vi "engUnitsToPulses.vi"(6 "Settings":T1, 7 "Channel":enum16{"X Axis", "Y Axis", "Z Axis"}(ring), 9 "Acceleration (mm/s^2)":dbl, 10 "Velocity (mm/s)":dbl, 11 "Position (mm)":dbl) -> (1 "kPulses /s^2":dbl, 2 "Pulses /s":dbl, 3 "Pulses":dbl)   [LabVIEW 2017]
uses:
  Settings/Settings-Control.ctl
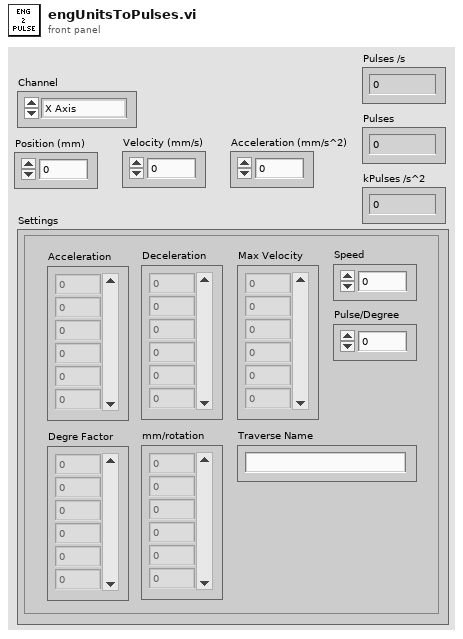
[diagram p1: front panel]
types:
  T1 = typedef "Settings-Control.ctl" = cluster{"Acceleration":dbl[], "Deceleration":dbl[], "Max Velocity":dbl[], "Speed":dbl, "Pulse/Degree":dbl, "Degre Factor":dbl[], "mm/rotation":dbl[], "Traverse Name":string}
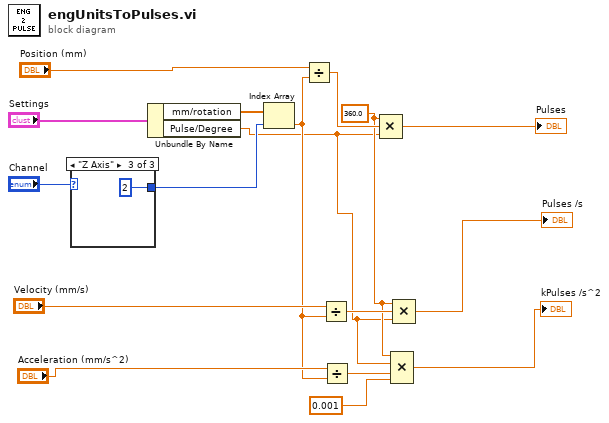
[diagram p0: block diagram]
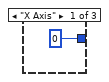
[diagram p2: hidden frame]
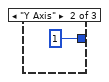
[diagram p3: hidden frame]
diagram:
  w5 = 360.0 ("x")
  n1 = case shown="\"Z Axis\"" "Channel" {
    tunnel: [0 1 2] -> w14
    frame "X Axis" {
    }
    frame "Y Axis" {
    }
    frame "Z Axis" {
    }
  }
  n2 = Unbundle By Name("Settings") -> ("mm/rotation"=w13:dbl[], "Pulse/Degree"=w4:dbl)
  n3 = Index Array(array=w13, index=w14) -> (element=w6:dbl)
  n4 = Divide(x="Position (mm)", y=w6) -> (x/y=w16:dbl)
  n5 = Divide(x="Velocity (mm/s)", y=w6) -> (x/y=w9:dbl)
  n6 = Divide(x="Acceleration (mm/s^2)", y=w6) -> (x/y=w3:dbl)
  n7 = Compound Arithmetic op=MULTIPLY(w5, w16, w4) -> (→"Pulses":dbl)
  n8 = Compound Arithmetic op=MULTIPLY(w5, w4, w3, 0.001 ("value")) -> (→"kPulses /s^2":dbl)
  n9 = Compound Arithmetic op=MULTIPLY(w5, w9, w4) -> (→"Pulses /s":dbl)
